vi "Import From File.vi"(8 "error in (no error)":errorcluster, 11 "Node Ptr":u64 format="%.0x") -> (0 "error out":errorcluster)   [LabVIEW 2013, in "MUX Custom Device.lvlib"]
uses:
  MUX Custom Device.lvlib
panel:
  in  "MUX Configuration Path":path
  in  "Cancel":bool
  in  "OK":bool
  in  "Tag":string
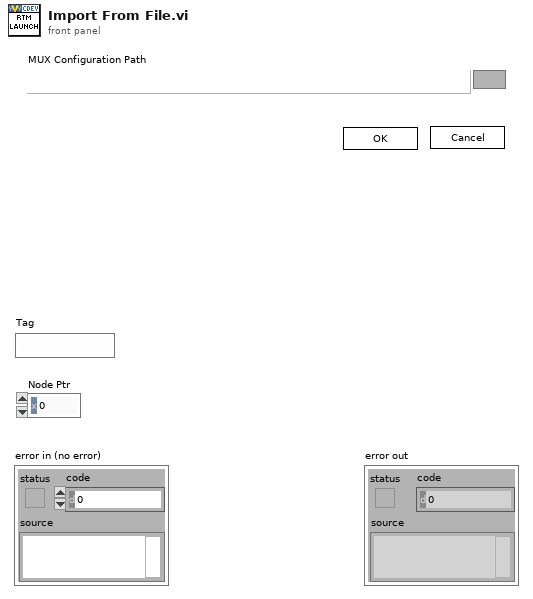
[diagram p1: front panel]
types:
  T1 = enum8{"Enabled", "Disabled", "Disabled and Grayed Out"}
  T2 = typedef "MUX Custom Device.lvlib/Mux Data.ctl" = cluster{"Mux Name":string, "Relay Channel Data":T3[]}
  T3 = typedef "MUX Custom Device.lvlib/Relay Channel Data.ctl" = cluster{"Relay Channel Name":string, "Relay Data":T4}
  T4 = typedef "MUX Custom Device.lvlib/Relay Data.ctl" = cluster{"Relay Name":string, "State":T5}
  T5 = typedef "MUX Custom Device.lvlib/Switch.ctl" = bool
  T6 = typedef "Custom Device API.lvlib/Custom Device Item Ref.ctl" = u64
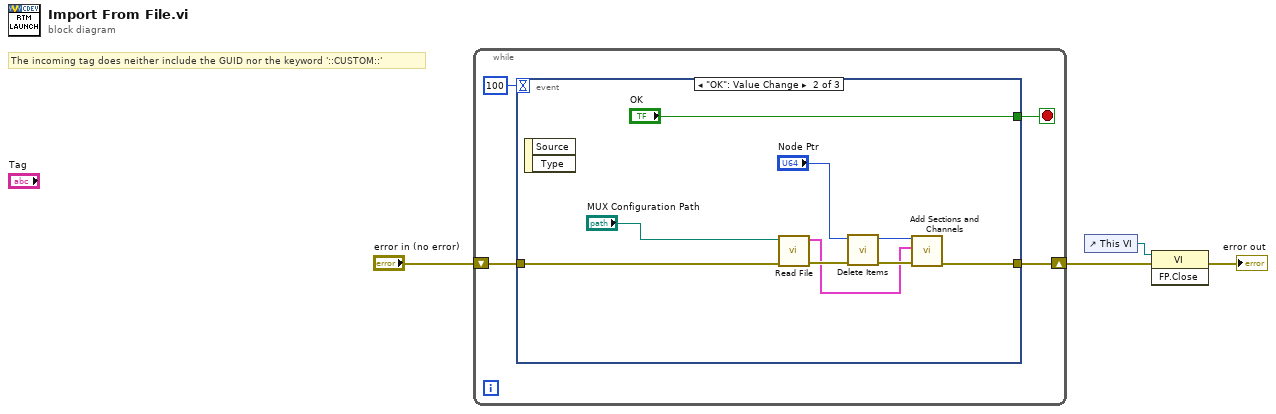
[diagram p0: block diagram]
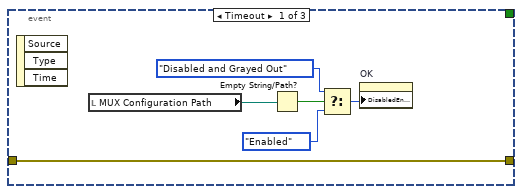
[diagram p2: hidden frame]
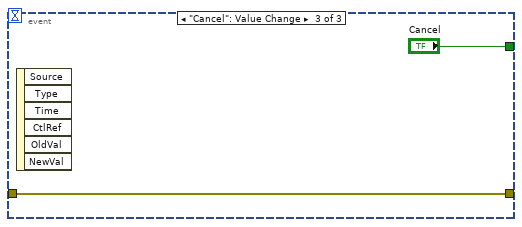
[diagram p3: hidden frame]
diagram:
  # "The incoming tag does neither include the GUID nor the keyword '::CUSTOM::'"
  n1 = while {
    shift-right: [w6] -> w2
    shift-left: "error in (no error)" -> [w7]
    stop <- w5 stop-if-true
    n2 = event shown="[1] \"OK\": Value Change" {
      selector: _ -> [_ _ _]
      dyn-events: _ -> [_ _ _]
      timeout: 100 -> [_ _ _]
      tunnel: w7 -> [w9 w22 w25]
      tunnel: [w9 w21 w25] -> w6
      tunnel: [_ "OK" "Cancel"] -> w5
      event Timeout {
        n3 = event-data() -> ()  [unwired: 1 in, 3 out]
        n4 = local read "MUX Configuration Path"() -> (w14:path)
        n5 = Empty String/Path?(string/path=w14) -> (empty?=w13:bool)
        n6 = Select(t=T1."Disabled and Grayed Out" ("Disabled"), s=w13, f=T1."Enabled" ("Disabled")) -> (s? t:f=w10:T1)
        n7 = property on="OK" class="Bool"("DisabledEnum"=w10) -> ()  [unwired: 2 in, 2 out]
      }
      event "OK": Value Change {
        n8 = event-data() -> ()  [unwired: 1 in, 2 out]
        n9 = call "Read File.vi"("Error In"=w22, "Mux File Path"="MUX Configuration Path") -> ("Error Out"=w18:errorcluster, "Mux Data Array"=w15:T2[])  [unwired: 8 in]
        n10 = call "Delete Items.vi"("error in (no error)"=w18, "Item Ref in"="Node Ptr") -> ("error out"=w19:errorcluster, "Item Ref out"=w16:T6)  [unwired: 8 in]
        n11 = call "Add Sections and Channels.vi"("Error In"=w19, "Mux Data Array"=w15, "Custom Device Ref in"=w16) -> ("Error Out"=w21:errorcluster)  [unwired: 7 in, 1 out]
      }
      event "Cancel": Value Change {
        n12 = event-data() -> ()  [unwired: 1 in, 6 out]
      }
    }
  }
  n13 = control-ref of="This VI"() -> (w3:refnum<vi>)
  n14 = invoke class="VI" method="FP.Close"(reference=w3, error in=w2) -> (error out=→"error out":errorcluster)  [unwired: 1 in, 2 out]
